vi "Wait For Current Play To Finish.vi"(8 "error in (no error)":errorcluster, 9 "Timeout (seconds) (Infinity)":dbl=inf, 11 "Sound Player in":refnum<class "Sound Player.lvclass">) -> (0 "error out":errorcluster, 3 "Sound Player out":refnum<class "Sound Player.lvclass">)   [LabVIEW 2017, in "Sound Player.lvclass"]
doc: "Wait for the sound currently playing on the player to complete. The default time out is \"Infinity\". Wiring a negative value will return an error."
uses:
  Sound Player.lvclass
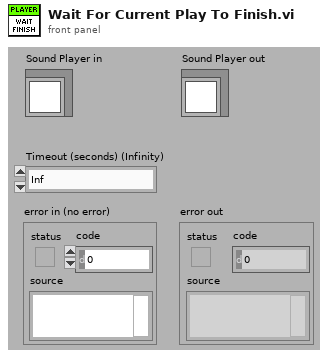
[diagram p1: front panel]
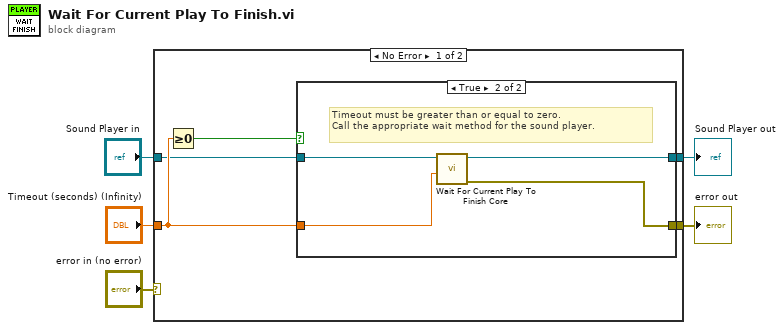
[diagram p0: block diagram]
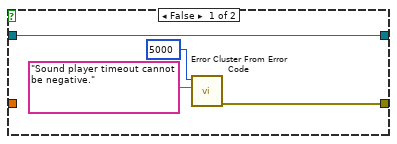
[diagram p2: hidden frame]
diagram:
  n1 = case shown="No Error" "error in (no error)" {
    selector: "error in (no error)" -> [_ w20]
    tunnel: [w9 w20] -> w4
    tunnel: [w6 w19] -> w2
    tunnel: "Sound Player in" -> [w7 w19]
    tunnel: "Timeout (seconds) (Infinity)" -> [w8 _]
    frame No Error {
      n2 = Greater Or Equal To 0?(x=w8) -> (x >= 0?=w10:bool)
      n3 = case shown="True" w10 {
        tunnel: [w12 w17] -> w9
        tunnel: w8 -> [_ w18]
        tunnel: w7 -> [w11 w16]
        tunnel: [w11 w15] -> w6
        frame False {
          n4 = call <vilib>:"Error Cluster From Error Code.vi"("error message (\"\")"="Sound player timeout cannot be negative." ("error message (\"\")"), "error code (0)"=5000) -> ("error out"=w12:errorcluster)  [unwired: 7 in]
        }
        frame True {
          # "Timeout must be greater than or equal to zero.\nCall the appropriate wait method for the sound player."
          n5 = call-dynamic "Wait For Current Play To Finish Core.vi"("Timeout (seconds) (Infinity)"=w18, "Sound Player in"=w16) -> ("error out"=w17:errorcluster, "Sound Player out"=w15:refnum<class "Sound Player.lvclass">)  [unwired: 8 in]
        }
      }
    }
    frame Error {
    }
  }
  "error out" <- w4
  "Sound Player out" <- w2
